vi "trigger_check_press.vi"(8 "error in (no error)":errorcluster, 9 "source":tag="/cDAQ4/PFI0", 10 "was_pressed?":bool, 11 "Refnum in":refnum<k21>) -> (0 "error out":errorcluster, 1 "is pressed?":bool, 3 "Refnum out":refnum<k21>)   [LabVIEW 2022 SP3]
uses:
  <vilib>/DAQmx/configure/trigger.llb/DAQmx Start Trigger (Digital Edge).vi
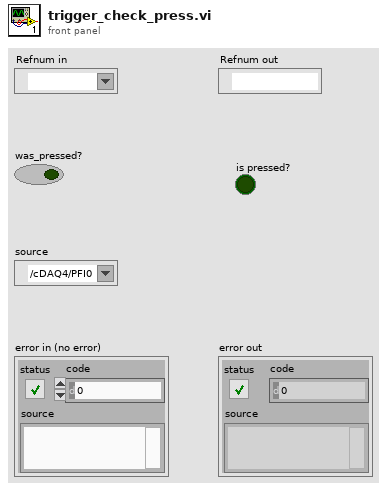
[diagram p1: front panel]
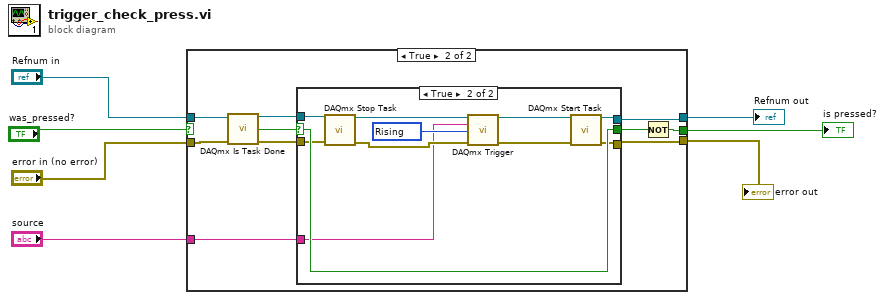
[diagram p0: block diagram]
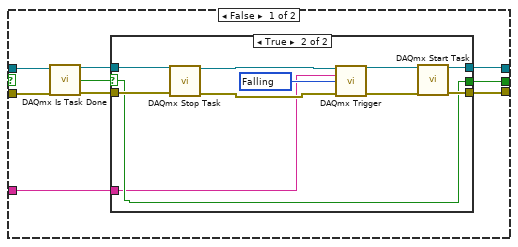
[diagram p2: hidden frame]
diagram:
  n1 = case shown="True" "was_pressed?" {
    tunnel: [w13 w40] -> w7
    tunnel: [w12 w36] -> w3
    tunnel: [w11 w34] -> w4
    tunnel: "Refnum in" -> [w10 w32]
    tunnel: "error in (no error)" -> [w9 w33]
    tunnel: "source" -> [w8 w31]
    frame False {
      n2 = call <vilib>:"DAQmx Is Task Done.vi"("task/channels in"=w10, "error in"=w9) -> ("task out"=w15:refnum<k21>, "task done?"=w16:bool, "error out"=w14:errorcluster)  [unwired: 11 in]
      n3 = case shown="True" w16 {
        selector: w16 -> [w17 w21]
        tunnel: w15 -> [w19 w25]
        tunnel: w14 -> [w18 w24]
        tunnel: [w17 w21] -> w13
        tunnel: [w19 w30] -> w12
        tunnel: [w18 w27] -> w11
        tunnel: w8 -> [_ w20]
        frame False {
        }
        frame True {
          w29 = 10171 items=["Rising"=10280, "Falling"=10171] ("edge")
          n4 = call <vilib>:"DAQmx Stop Task.vi"("task/channels in"=w25, "error in"=w24) -> ("task out"=w22:refnum<k21>, "error out"=w23:errorcluster)  [unwired: 12 in]
          n5 = call-poly <vilib>:"DAQmx Trigger.vi"("task/channels in"=w22, "source"=w20, "edge"=w29, "error in"=w23) -> ("task out"=w28:refnum<k21>, "error out"=w26:errorcluster)  [unwired: 10 in]
          n6 = call <vilib>:"DAQmx Start Task.vi"("task/channels in"=w28, "error in"=w26) -> ("task out"=w30:refnum<k21>, "error out"=w27:errorcluster)  [unwired: 12 in]
        }
      }
    }
    frame True {
      n7 = call <vilib>:"DAQmx Is Task Done.vi"("task/channels in"=w32, "error in"=w33) -> ("task out"=w37:refnum<k21>, "task done?"=w39:bool, "error out"=w35:errorcluster)  [unwired: 11 in]
      n8 = case shown="True" w39 {
        selector: w39 -> [w43 w53]
        tunnel: [w43 w53] -> w38
        tunnel: [w42 w50] -> w36
        tunnel: w37 -> [w42 w46]
        tunnel: w35 -> [w41 w45]
        tunnel: [w41 w49] -> w34
        tunnel: w31 -> [_ w44]
        frame False {
        }
        frame True {
          w54 = 10280 items=["Rising"=10280, "Falling"=10171] ("edge")
          n9 = call <vilib>:"DAQmx Stop Task.vi"("task/channels in"=w46, "error in"=w45) -> ("task out"=w47:refnum<k21>, "error out"=w48:errorcluster)  [unwired: 12 in]
          n10 = call-poly <vilib>:"DAQmx Trigger.vi"("task/channels in"=w47, "source"=w44, "edge"=w54, "error in"=w48) -> ("task out"=w52:refnum<k21>, "error out"=w51:errorcluster)  [unwired: 10 in]
          n11 = call <vilib>:"DAQmx Start Task.vi"("task/channels in"=w52, "error in"=w51) -> ("task out"=w50:refnum<k21>, "error out"=w49:errorcluster)  [unwired: 12 in]
        }
      }
      n12 = Not(x=w38) -> (.not. x?=w40:bool)
    }
  }
  "is pressed?" <- w7
  "error out" <- w4
  "Refnum out" <- w3
